vi "Read From Console.vi"(8 "error in (no error)":errorcluster caption="错误输入（无错误）") -> (0 "error out":errorcluster caption="错误输出", 3 "Output":string)   [LabVIEW 2013]
doc: "该模板用于创建子VI。"
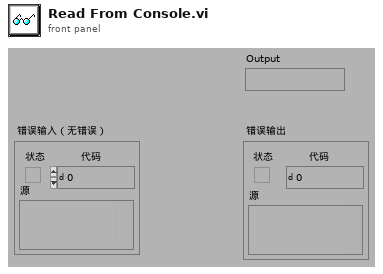
[diagram p1: front panel]
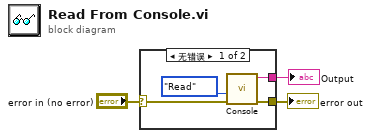
[diagram p0: block diagram]
diagram:
  n1 = case shown="无错误" "error in (no error)" {
    selector: "error in (no error)" -> [w7 w8]
    tunnel: [w6 w8] -> w2
    tunnel: [w4 _] -> w1
    frame No Error {
      n2 = call "Console.vi"("error in (no error)"=w7, "Mode"=enum16{"Write", "Read", "Clear"}."Read") -> ("error out"=w6:errorcluster, "Output"=w4:string)  [unwired: 8 in]
    }
    frame Error {
    }
  }
  "error out" <- w2
  "Output" <- w1
